vi "get channels.vi"(11 "PID Module 2 configuration in":refnum<class "PID Module 2 configuration.lvclass">) -> (2 "channels":refnum<class "TBM channel.lvclass">[](array[class]), 3 "PID Module 2 configuration out":refnum<class "PID Module 2 configuration.lvclass">)   [LabVIEW 2015, in "PID Module 2 configuration.lvclass"]
doc: "Returns an array of all Channels currently added to this configuration object."
uses:
  PID Module 2 configuration.lvclass
  <vilib>/NI/Tag Bus Module Framework/channel/TBM channel.lvclass
  PID Module 2 configuration.lvclass/PID Module 2 configuration.ctl
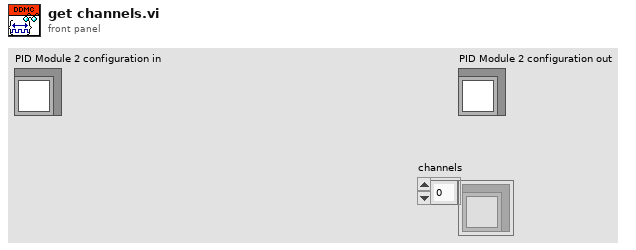
[diagram p1: front panel]
types:
  T1 = typedef "PID Module 2 configuration.lvclass/Line.ctl" = cluster{"PID ID":string, "Setpoint":refnum<class "TBM channel.lvclass">, "Variable":refnum<class "TBM channel.lvclass">, "Output":refnum<class "TBM channel.lvclass">, "Output High":refnum<class "TBM channel.lvclass">, "Output Low":refnum<class "TBM channel.lvclass">, "P":refnum<class "TBM channel.lvclass">, "I":refnum<class "TBM channel.lvclass">, "D":refnum<class "TBM channel.lvclass">}
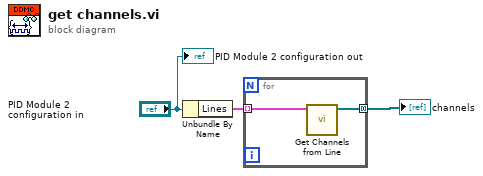
[diagram p0: block diagram]
diagram:
  n1 = Unbundle By Name("PID Module 2 configuration in") -> ("Lines"=w2:T1[])
  n2 = for {
    tunnel: w2 -> [w5] mode=indexing
    tunnel: [w4] -> w1 mode=concatenating
    n3 = call "Get Channels from Line.vi"("Line"=w5) -> ("Channels"=w4:refnum<class "TBM channel.lvclass">[])  [unwired: 10 in]
  }
  "channels" <- w1
  "PID Module 2 configuration out" <- "PID Module 2 configuration in"
